vi "Mask Control.vi"(2 "Image Src":T1, 4 "Rectangle Mask":i32[](array[numeric]), 5 "error in (no error)":errorcluster) -> (7 "Image Dst Out":T1, 9 "error out":errorcluster)   [LabVIEW 2011]
uses:
  <vilib>/vision/Image Controls.llb/IMAQ Image.ctl
  <vilib>/vision/NI_Vision_Development_Module.lvlib
panel:
  # "This VI applies a mask to the incoming image.\nPractically, it just crops the image to a region of interest.\nUsed to increase image processing speed by reducing area to search.\n\n\"Focus\" is an option that uses the location data of the targeted rectange\nfrom the previous loop iteration to use a tighter mask for additional \nprocessing speed."
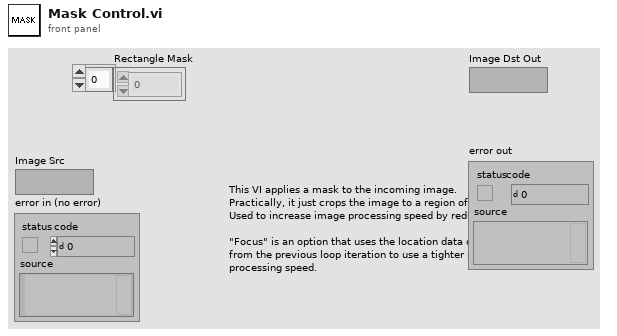
[diagram p1: front panel]
types:
  T1 = typedef "IMAQ Image.ctl" = refnum<image>
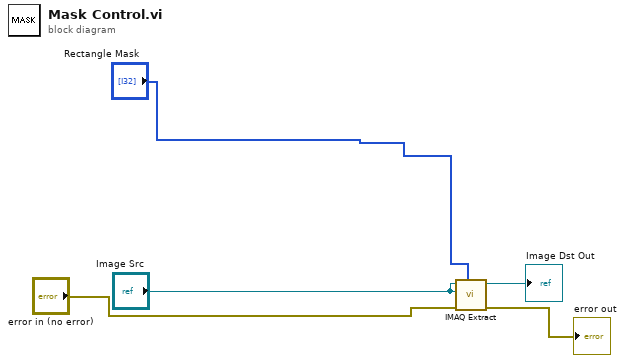
[diagram p0: block diagram]
diagram:
  n1 = call "IMAQ Extract"("Optional Rectangle"="Rectangle Mask", "error in (no error)"="error in (no error)", "Image Dst"="Image Src", "Image Src"="Image Src") -> ("error out"=→"error out":errorcluster, "Image Dst Out"=→"Image Dst Out":T1)  [unwired: 6 in]
